vi "galvo.vi"() -> ()   [LabVIEW 2017]
panel:
  in  "fixed y":dbl
  in  "fixed x":dbl
  in  "mode":u16(ring) items=["oscillate", "grid"]
  in  "genstop":bool
  in  "oscillate X":bool=TRUE
  in  "oscillate Y":bool=TRUE
  in  "stop":bool
  # "GALVO"
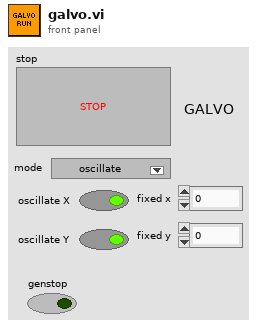
[diagram p1: front panel]
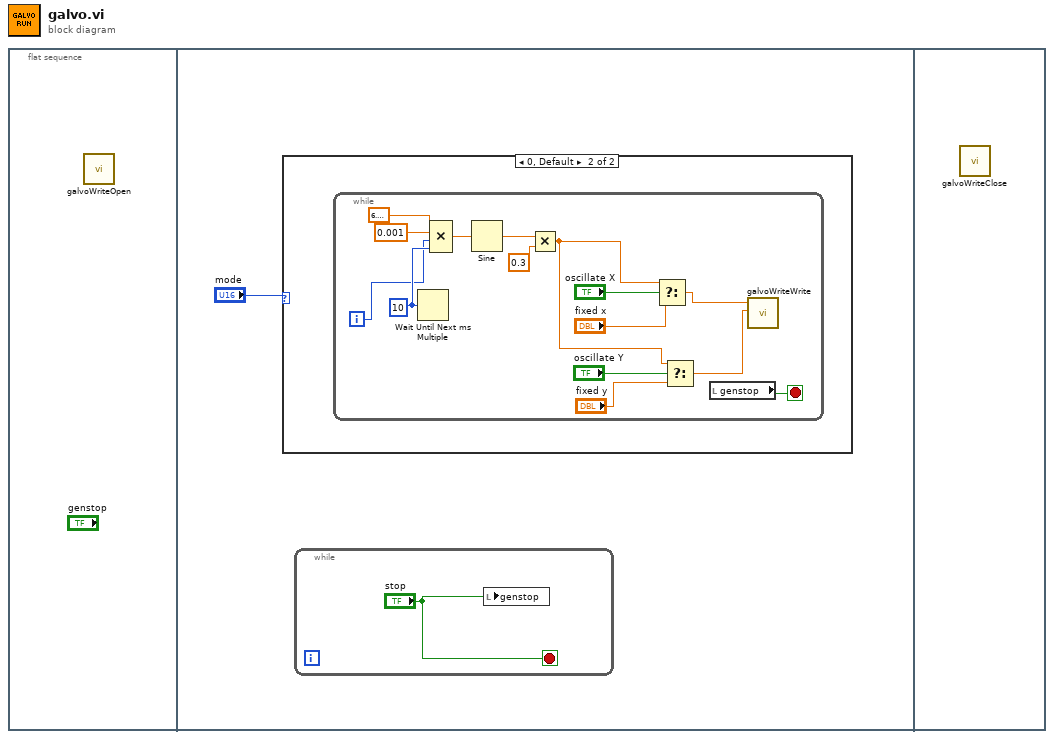
[diagram p0: block diagram]
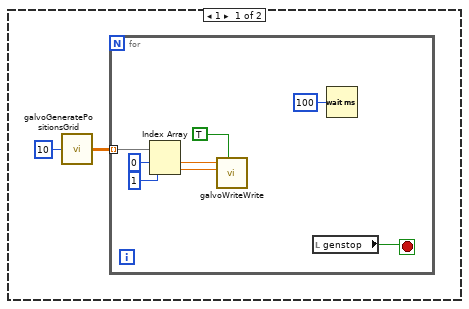
[diagram p2: hidden frame]
diagram:
  n1 = flat-sequence {
    frame #0 {
      n2 = call "galvoWriteOpen.vi"() -> ()  [unwired: 12 in]
    }
    frame #1 {
      n3 = case shown="0, Default" "mode" {
        frame 1 {
          n4 = call "galvoGeneratePositionsGrid.vi"("N-1"=10) -> ("grid"=w3:dbl[][])
          n5 = for {
            tunnel: w3 -> [w12] mode=indexing
            stop <- w5 stop-if-true
            n6 = Index Array(array=w12, index #1=0 ("index"), index #2=1 ("index")) -> (element #1=w9:dbl, element #2=w8:dbl)
            n7 = call "galvoWriteWrite.vi"("X"=w9, "Y"=w8, "fractional units (T)"=TRUE) -> ()  [unwired: 3 in]
            n8 = local read "genstop"() -> (w5:bool)
            n9 = Wait (ms)(milliseconds to wait=u32 100) -> ()  [unwired: 1 out]
          }
        }
        frame 0, Default {
          n10 = while {
            i -> [w24]
            stop <- w20 stop-if-true
            w25 = u32 10 ("millisecond multiple")
            n11 = Wait Until Next ms Multiple(millisecond multiple=w25) -> ()  [unwired: 1 out]
            n12 = Compound Arithmetic op=MULTIPLY(6.283185307179586, 0.001 ("value"), w24, w25) -> (w23:dbl)
            n13 = Sine(x=w23) -> (sin(x)=w22:dbl)
            n14 = Multiply(x=w22, y=0.3) -> (x*y=w16:dbl)
            n15 = Select(t=w16, s="oscillate X", f="fixed x") -> (s? t:f=w14:dbl)
            n16 = Select(t=w16, s="oscillate Y", f="fixed y") -> (s? t:f=w13:dbl)
            n17 = local read "genstop"() -> (w20:bool)
            n18 = call "galvoWriteWrite.vi"("X"=w14, "Y"=w13) -> ()  [unwired: 4 in]
          }
        }
      }
      n19 = while {
        stop <- "stop" stop-if-true
        n20 = local write "genstop"("stop") -> ()
      }
    }
    frame #2 {
      n21 = call "galvoWriteClose.vi"() -> ()  [unwired: 12 in]
    }
  }
